vi "Reinitialize.vi"(8 "error in (no error)":errorcluster, 11 "VISA resource name":refnum<visa-resource-name>="COM4") -> (0 "error out":errorcluster, 3 "VISA resource name out":refnum<visa-resource-name>)   [LabVIEW 2017]
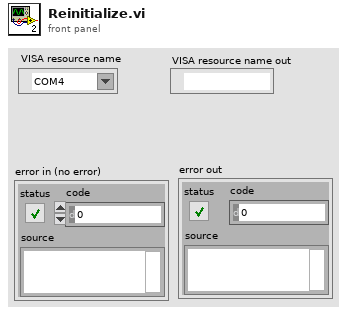
[diagram p1: front panel]
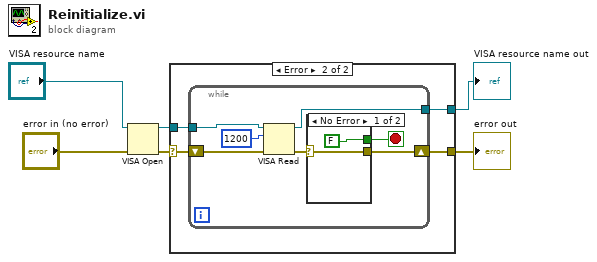
[diagram p0: block diagram]
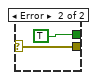
[diagram p3: hidden frame]
diagram:
  n1 = VISA Open(error in (no error)="error in (no error)", VISA resource name="VISA resource name") -> (VISA resource name=w1:refnum<visa-resource-name>, error out=w4:errorcluster)  [unwired: 3 in]
  n2 = case shown="Error" w4 {
    selector: w4 -> [w7 w12]
    tunnel: [w8 w9] -> w3
    tunnel: [w7 w11] -> w2
    tunnel: w1 -> [w8 w10]
    frame No Error {
    }
    frame Error {
      n3 = while {
        shift-right: [w16] -> w11
        shift-left: w12 -> [w18]
        tunnel: w10 -> [w15]
        tunnel: [w14] -> w9
        stop <- w13 stop-if-true
        n4 = VISA Read(VISA resource name=w15, byte count=u32 1200, error in (no error)=w18) -> (VISA resource name out=w14:refnum<visa-resource-name>, error out=w17:errorcluster)  [unwired: 2 out]
        n5 = case shown="No Error" w17 {
          selector: w17 -> [w21 w23]
          tunnel: [w21 w23] -> w16
          tunnel: [FALSE TRUE] -> w13
          frame No Error {
          }
          frame Error {
          }
        }
      }
    }
  }
  "error out" <- w2
  "VISA resource name out" <- w3
